vi "Oxford Merc PS Get Field.vi"(8 "Error In":errorcluster, 11 "VISA resource name":refnum<visa-resource-name>="tcpip::192.168.1.28::7020::socket") -> (0 "Error Out":errorcluster, 2 "Magnetic Field (T)":dbl, 3 "VISA resource name out":refnum<visa-resource-name>)   [LabVIEW 2019]
panel:
  out "Response 2":string
  out "Response":string
  out "AtoB":dbl caption="Current Field Factor (A/T)" format="%#.1f"
  out "Current":dbl
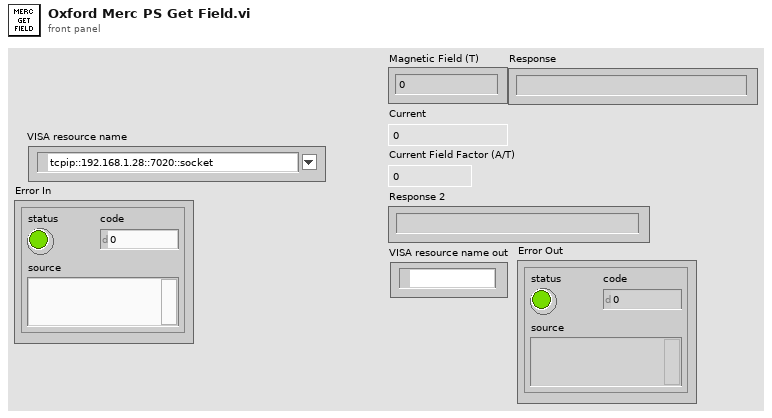
[diagram p1: front panel]
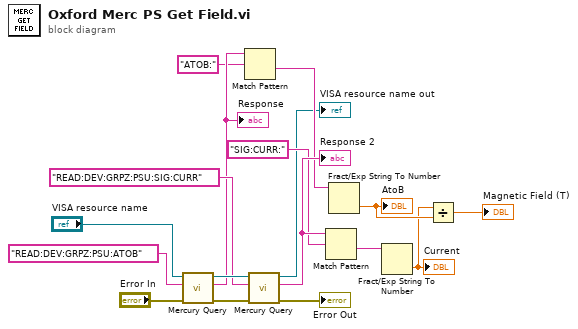
[diagram p0: block diagram]
diagram:
  n1 = call "Mercury Query.vi"("Error In"="Error In", "Command"="READ:DEV:GRPZ:PSU:ATOB", "VISA resource name"="VISA resource name") -> ("Error Out"=w14:errorcluster, "Response"=w11:string, "VISA resource name out"=w13:refnum<visa-resource-name>)  [unwired: 6 in]
  "Response" <- w11
  n2 = Match Pattern(string=w11, regular expression="ATOB:") -> (after substring=w7:string)  [unwired: 1 in, 3 out]
  n3 = call "Mercury Query.vi"("Error In"=w14, "Command"="READ:DEV:GRPZ:PSU:SIG:CURR", "VISA resource name"=w13) -> ("Error Out"=→"Error Out":errorcluster, "Response"=w9:string, "VISA resource name out"=→"VISA resource name out":refnum<visa-resource-name>)  [unwired: 6 in]
  "Response 2" <- w9
  n4 = Match Pattern(string=w9, regular expression="SIG:CURR:") -> (after substring=w5:string)  [unwired: 1 in, 3 out]
  n5 = Fract/Exp String To Number(string=w7) -> (number=w6:dbl)  [unwired: 3 in, 1 out]
  "AtoB" <- w6
  n6 = Fract/Exp String To Number(string=w5) -> (number=w4:dbl)  [unwired: 3 in, 1 out]
  "Current" <- w4
  n7 = Divide(x=w4, y=w6) -> (x/y=→"Magnetic Field (T)":dbl)
